vi "Exec.vi"(3 "Commands in":string) -> (1 "Commands out":string)   [LabVIEW 2012]
uses:
  <vilib>/regexp/Match Regular Expression.xnode
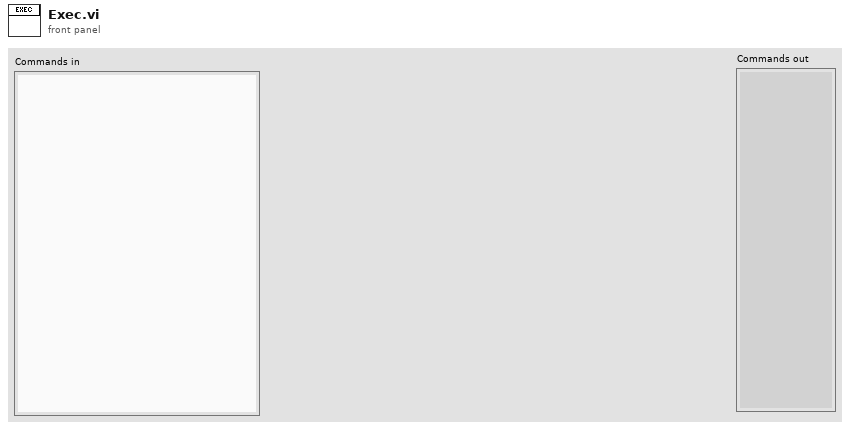
[diagram p1: front panel]
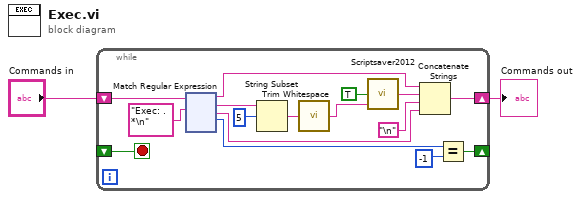
[diagram p0: block diagram]
diagram:
  n1 = while {
    shift-right: [w11] -> w1
    shift-left: "Commands in" -> [w17]
    shift-right: [w4] -> _
    shift-left: _ -> [w3]
    stop <- w3 stop-if-true
    n2 = xnode "Match Regular Expression"("input string"=w17, "regular expression"="Exec: .*\n") -> ("before match"=w13:string, "whole match"=w16:string, "after match"=w8:string, "offset past match"=w6:i32)  [unwired: 4 in, 1 out]
    n3 = String Subset(string=w16, offset (0)=5) -> (substring=w10:string)  [unwired: 1 in]
    n4 = call <vilib>:"Trim Whitespace.vi"("string"=w10) -> ("trimmed string"=w9:string)  [unwired: 1 in]
    n5 = call "Scriptsaver2012.vi"("Filename"=w9, "Save (0)/Load (1)"=TRUE) -> ("Loaded Script"=w12:string)  [unwired: 1 in]
    n6 = Concatenate Strings(w13, w12, "\n", w8) -> (w11:string)
    n7 = Equal?(x=w6, y=-1) -> (x = y?=w4:bool)
  }
  "Commands out" <- w1
